vi "Connect.vi"(8 "error in (no error)":errorcluster, 10 "Connection list in":string, 11 "SLSC Switch Consumer in":refnum<class "NI-SWITCH Consumer.lvclass">=refnum) -> (0 "error out":errorcluster, 3 "SLSC Switch Consumer out":refnum<class "NI-SWITCH Consumer.lvclass">)   [LabVIEW 2017, in "NI-SWITCH Messaging.lvlib" / "NI-SWITCH Consumer.lvclass"]
uses:
  NI-SWITCH Consumer.lvclass
  NI-SWITCH Consumer.lvclass/NI-SWITCH Consumer.ctl
  <vilib>/SLSC_Switch/Connect Channels (Multiple).vi
  <vilib>/SLSC_Switch/SLSC Switch.lvlib
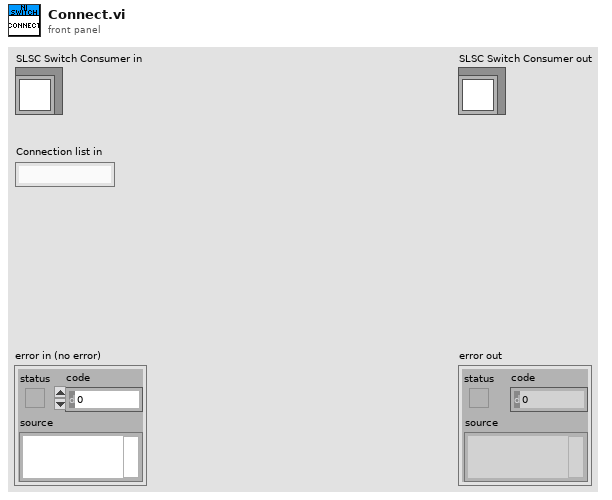
[diagram p1: front panel]
types:
  T1 = typedef "nislscslSession.ctl" = refnum<k20>
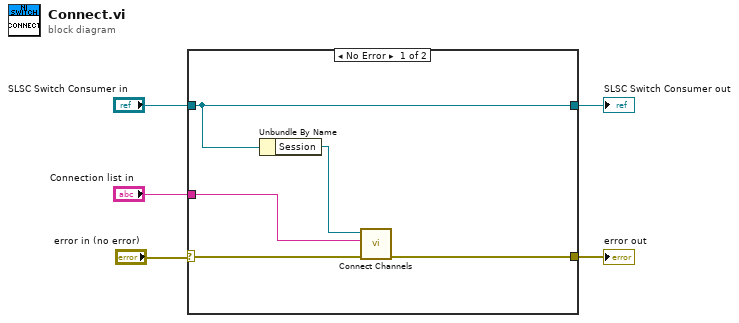
[diagram p0: block diagram]
diagram:
  n1 = case shown="No Error" "error in (no error)" {
    selector: "error in (no error)" -> [w7 w12]
    tunnel: [w6 w12] -> w4
    tunnel: [w10 w11] -> w1
    tunnel: "SLSC Switch Consumer in" -> [w10 w11]
    tunnel: "Connection list in" -> [w8 _]
    frame No Error {
      n2 = Unbundle By Name(w10) -> ("Session"=w9:T1)
      n3 = call-poly <vilib>:"Connect Channels.vi"("error in (no error)"=w7, "connection list"=w8, "session in"=w9) -> ("error out"=w6:errorcluster)  [unwired: 7 in, 1 out]
    }
    frame Error {
    }
  }
  "error out" <- w4
  "SLSC Switch Consumer out" <- w1
